vi "get refs from dvr.vi"() -> (2 "Controls":refnum<vi>[](array[refnum]))   [LabVIEW 2018]
uses:
  class1/TypeDef/Data.ctl
  class1/TypeDef/Settings.ctl
  <vilib>/Utility/traverseref.llb/TRef TravTarget.ctl
  <vilib>/Utility/traverseref.llb/VI Scripting - Traverse.lvlib
  class1/class1.lvclass
panel:
  out "error out 2":errorcluster
  out "Array 2":string[](array[string])
  out "Label.Text":string
  out "Array":string[](array[string])
  in  "Tree":string(tree)
  in  "DVR":refnum<data-value>
  out "error out":errorcluster
  in  "error in (no error)":errorcluster
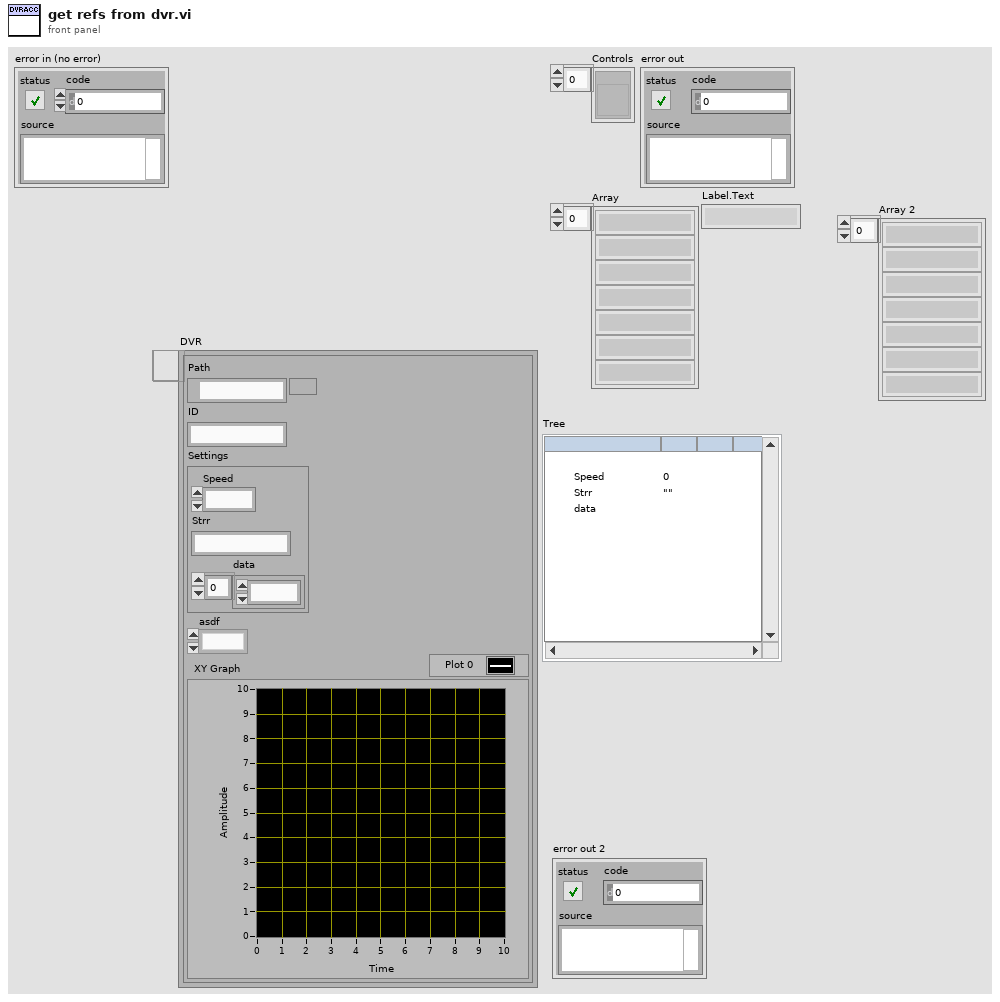
[diagram p1: front panel]
types:
  T1 = typedef "class1.lvclass/Settings.ctl" = cluster{"Speed":dbl, "Strr":string, "data":i32[]}
  T2 = typedef "TRef TravTarget.ctl" = enum16{"FP", "BD", "Other"}
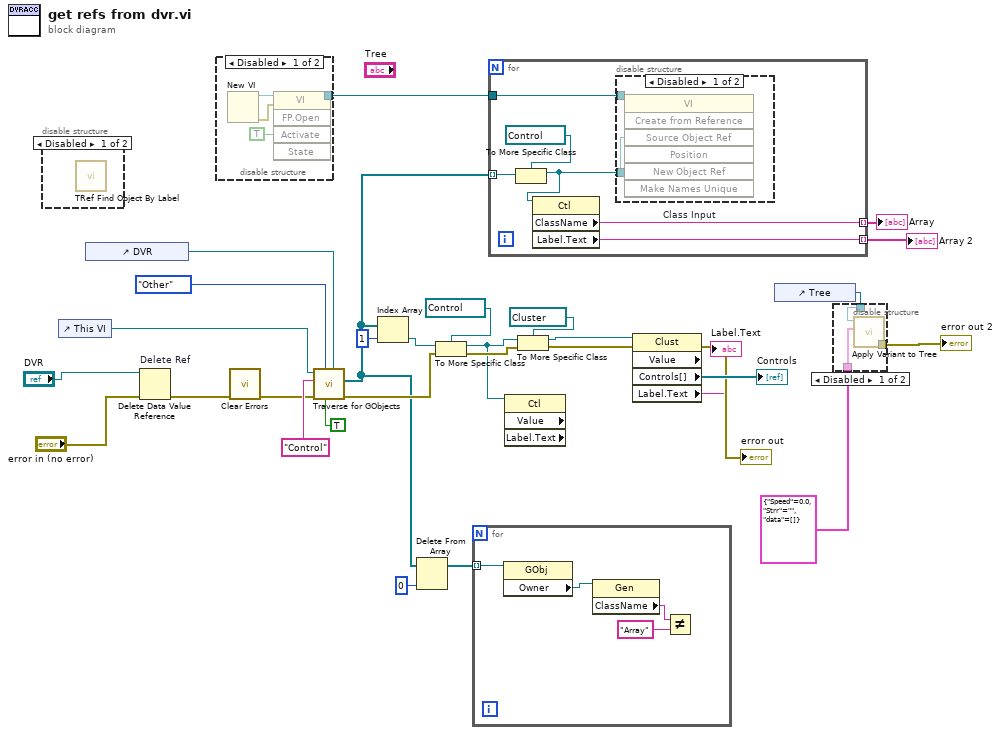
[diagram p0: block diagram]
diagram:
  n1 = disable-structure shown="Disabled" {
    frame Disabled {
      n2 = call <vilib>:"TRef Find Object By Label.vi"() -> ()  [unwired: 8 in, 4 out]
    }
    frame Enabled {
    }
  }
  n3 = control-ref of="This VI"() -> (w19:refnum<vi>)
  n4 = control-ref of="DVR"() -> (w15:refnum<vi>)
  n5 = Delete Data Value Reference "Delete Ref"(data value reference="DVR", error in="error in (no error)") -> (error out=w23:errorcluster)  [unwired: 1 out]
  n6 = disable-structure shown="Disabled" {
    disable-tunnel: [w31 _] -> w16
    frame Disabled {
      n7 = New VI() -> (0:w33:errorcluster, 3:w34:refnum<vi>)  [unwired: 7 in]
      n8 = invoke class="VI" method="FP.Open"(reference=w34, error in=w33, "Activate"=TRUE ("Activate?")) -> (reference out=w31:refnum<vi>)  [unwired: 2 in, 4 out]
    }
    frame Enabled {
    }
  }
  n9 = call <vilib>:"Clear Errors.vi"("error in (no error)"=w23) -> ("error out"=w17:errorcluster)  [unwired: 5 in, 1 out]
  n10 = call <vilib>:"Traverse for GObjects.vi"("Other Refnum"=w15, "Traverse Generated Code (F)"=TRUE, "Traverse Target"=TRef_TravTarget."Other", "error in (no error)"=w17, "Class Name"="Control", "VI Refnum"=w19) -> ("error out"=w9:errorcluster, "References"=w3:refnum<vi>[])  [unwired: 2 in, 2 out]
  n11 = Index Array(array=w3, index=1) -> (element=w12:refnum<vi>)
  n12 = Delete From Array(array=w3, index=0) -> (array with subset deleted=w1:refnum<vi>[])  [unwired: 1 in, 1 out]
  n13 = To More Specific Class(target class=refnum<vi> refnum ("Source Object Reference"), reference=w12, error in=w9) -> (specific class reference=w6:refnum<vi>, error out=w10:errorcluster)
  n14 = for {
    tunnel: w1 -> [w38] mode=indexing
    n15 = property class="GObj"(reference=w38) -> ("Owner"=w37:refnum<vi>)  [unwired: 1 in, 2 out]
    n16 = property class="Gen"(reference=w37) -> ("ClassName"=w36:string)  [unwired: 1 in, 2 out]
    n17 = Not Equal?(x=w36, y="Array") -> ()  [unwired: 1 out]
  }
  n18 = for {
    tunnel: w3 -> [w42] mode=indexing
    tunnel: [w44] -> w13 mode=indexing
    tunnel: w16 -> [w43]
    tunnel: [w39] -> w7 mode=indexing
    n19 = To More Specific Class(target class=refnum<vi> refnum ("Source Object Reference"), reference=w42) -> (specific class reference=w40:refnum<vi>)  [unwired: 1 in, 1 out]
    n20 = property class="Ctl"(reference=w40) -> ("ClassName"=w44:string, "Label.Text"=w39:string)  [unwired: 1 in, 2 out]
    n21 = disable-structure shown="Disabled" {
      disable-tunnel: w43 -> [w46 _]
      disable-tunnel: w40 -> [w45 _]
      frame Disabled {
        n22 = invoke on="Class Input" class="VI" method="Create from Reference"(reference=w46, "Source Object Ref"=w45) -> ()  [unwired: 5 in, 7 out]
      }
      frame Enabled {
      }
    }
  }
  "Array" <- w13
  "Array 2" <- w7
  n23 = property class="Ctl" props=["Value", "Label", "Text"](reference=w6) -> ()  [unwired: 1 in, 4 out]
  n24 = To More Specific Class(target class=refnum<vi> refnum ("Numeric"), reference=w6, error in=w10) -> (specific class reference=w25:refnum<vi>, error out=w24:errorcluster)
  n25 = property class="Clust" props=["Value", "Controls[]", "Label", "Text"](reference=w25, error in=w24) -> (error out=→"error out":errorcluster, "Controls[]"=→"Controls":refnum<vi>[], "Label.Text"=→"Label.Text":string)  [unwired: 2 out]
  n26 = control-ref of="Tree"() -> (w14:refnum<vi>)
  n27 = disable-structure shown="Disabled" {
    disable-tunnel: w14 -> [w49 _]
    disable-tunnel: [w48 _] -> w5
    disable-tunnel: T1 {"Speed"=0.0, "Strr"="", "data"=[]} ("Settings") -> [w47 _]
    frame Disabled {
      n28 = call <vilib>:"Apply Variant to Tree.vi"("Variant"=w47, "TreeControl in"=w49) -> ("error out"=w48:errorcluster)  [unwired: 8 in, 1 out]
    }
    frame Enabled {
    }
  }
  "error out 2" <- w5
